vi "testCount.vi"(8 "error in (no error)":errorcluster, 11 "TestCase in":refnum<class "ListImp_Common.lvclass">) -> (0 "error out":errorcluster, 3 "TestCase out":refnum<class "ListImp_Common.lvclass">)   [LabVIEW 2013, in "ListImp_Common.lvclass"]
uses:
  ListImp_Common.lvclass
  ListImp_Common.lvclass/ListImp_Common.ctl
  source/LapDog.Collections.Lists/ListImp/ListImp.lvclass
  <vilib>/addons/_JKI Toolkits/VI Tester/TestCase.llb/TestCase.lvclass
  UnitTestComparisons/UnitTestComparisons.lvlib
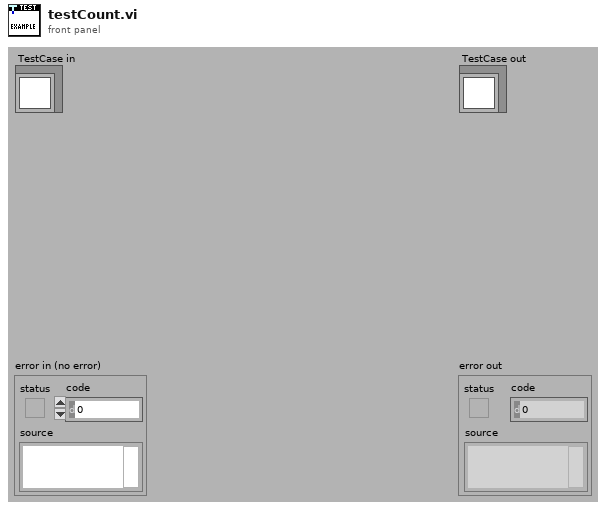
[diagram p1: front panel]
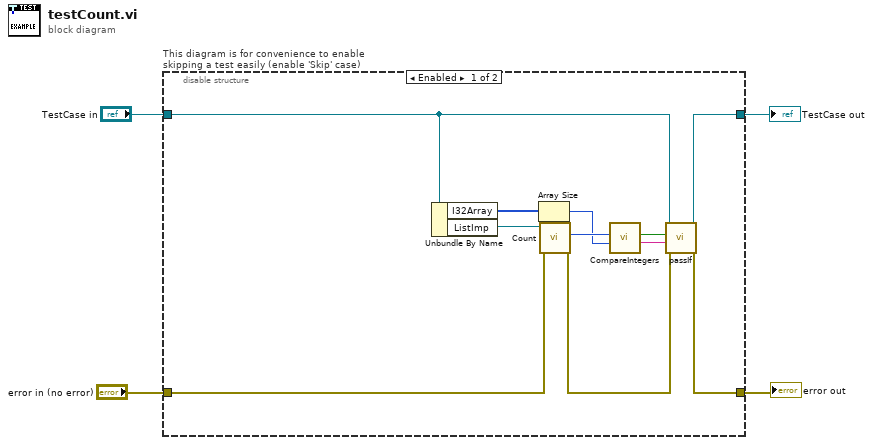
[diagram p0: block diagram]
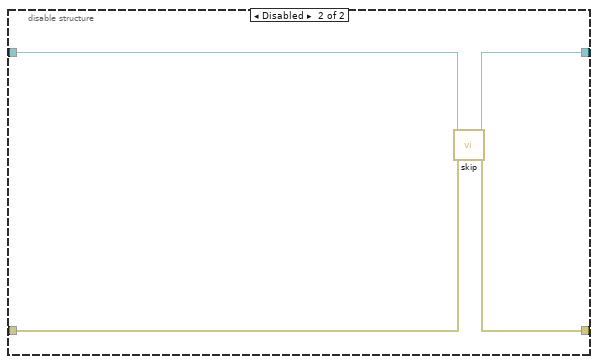
[diagram p2: hidden frame]
diagram:
  n1 = disable-structure "This diagram is for convenience to enable skipping a test easily (enable 'Skip' case)" shown="Enabled" {
    disable-tunnel: "TestCase in" -> [w13 w19]
    disable-tunnel: [w15 w17] -> w1
    disable-tunnel: [w14 w18] -> w3
    disable-tunnel: "error in (no error)" -> [w8 w16]
    frame Enabled {
      n2 = Unbundle By Name(w13) -> ("I32Array"=w6:i32[], "ListImp"=w10:refnum<class "ListImp.lvclass">)
      n3 = Array Size(array=w6) -> (size(s)=w5:i32)
      n4 = call-dynamic "Count.vi"("error in (no error)"=w8, "ListImp in"=w10) -> ("error out"=w7:errorcluster, "Number of Items"=w9:i32)  [unwired: 7 in, 1 out]
      n5 = call "CompareIntegers.vi"("Expected Value"=w5, "Actual Value"=w9) -> ("Message"=w11:string, "Equal?"=w12:bool)  [unwired: 8 in]
      n6 = call-dynamic "passIf.vi"("error in (no error)"=w7, "message (\"\")"=w11, "pass"=w12, "TestCase in"=w13) -> ("error out"=w14:errorcluster, "TestCase out"=w15:refnum<class "ListImp_Common.lvclass">)  [unwired: 6 in]
    }
    frame Disabled {
      # "skip test result while test is under development"
      n7 = call <vilib>:"skip.vi"("error in (no error)"=w16, "TestCase in"=w19) -> ("error out"=w18:errorcluster, "TestCase out"=w17:refnum<class "ListImp_Common.lvclass">)  [unwired: 8 in]
    }
  }
  "error out" <- w3
  "TestCase out" <- w1
